vi "Retrieve Airmar Data.vi"(11 "tCRD in":refnum<class "Aircraft OPCCRD.lvclass">) -> (0 "error out":errorcluster, 3 "tCRD out":refnum<class "Aircraft OPCCRD.lvclass">)   [LabVIEW 2015, in "Aircraft OPCCRD.lvclass"]
uses:
  Aircraft OPCCRD.lvclass
  Data/tCRD Data.lvclass
  Reusable/CRDS/Main/CRDS.lvclass
  Reusable/CRDS/Data/Main/CRDS Data.lvclass
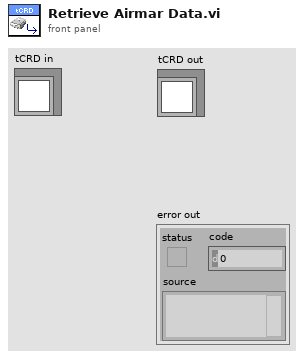
[diagram p1: front panel]
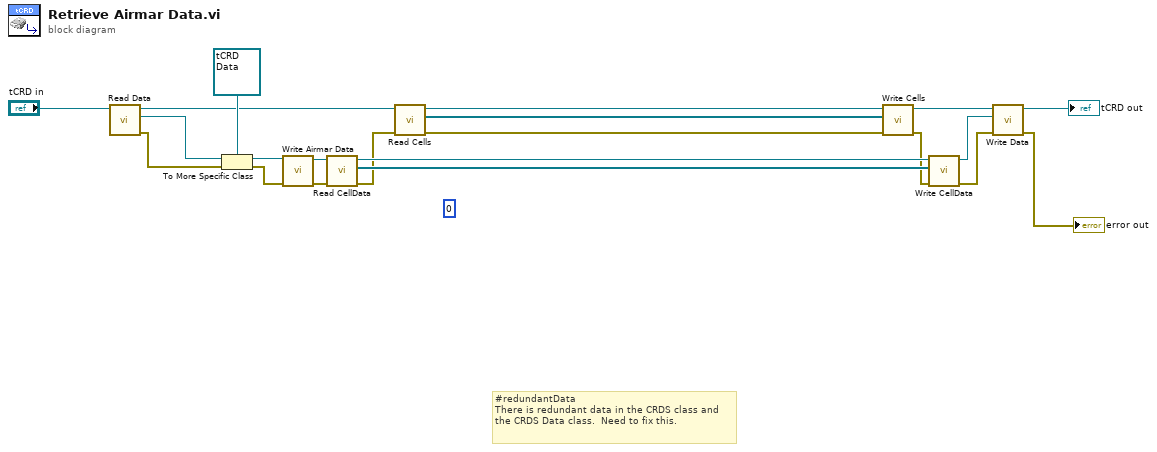
[diagram p0: block diagram]
diagram:
  (unwired) 0
  # "#redundantData\nThere is redundant data in the CRDS class and the CRDS Data class.  Need to fix this."
  n1 = call "Read Data.vi"("CRDS in"="tCRD in") -> ("error out"=w15:errorcluster, "CRDS"=w20:refnum<class "CRDS Data.lvclass">, "CRDS out"=w13:refnum<class "Aircraft OPCCRD.lvclass">, "error in (no error)"=w14:errorcluster)  [unwired: 7 in]
  n2 = To More Specific Class(target class=refnum<class "tCRD Data.lvclass"> refnum ("tCRD Data"), reference=w20, error in=w15) -> (specific class reference=w18:refnum<class "tCRD Data.lvclass">, error out=w17:errorcluster)
  n3 = call "Write Airmar Data.vi"("error in (no error)"=w17, "tCRD Data in"=w18) -> ("error out"=w4:errorcluster, "tCRD Data out"=w8:refnum<class "tCRD Data.lvclass">, "Airmar Data"=w16:refnum<class "Airmar Data.lvclass">)  [unwired: 7 in]
  n4 = call "Read CellData.vi"("error in"=w4, "CRDS Data in"=w8) -> ("error out"=w5:errorcluster, "CellData"=w6:refnum<class "CRDS Cell Data.lvclass">[], "CRDS Data out"=w7:refnum<class "tCRD Data.lvclass">)  [unwired: 7 in]
  n5 = call "Read Cells.vi"("error in (no error)"=w5, "CRDS in"=w13) -> ("error out"=w2:errorcluster, "Cells"=w10:refnum<class "CRDS Cell.lvclass">[], "CRDS out"=w12:refnum<class "Aircraft OPCCRD.lvclass">)  [unwired: 7 in]
  n6 = call "Write Cells.vi"("error in (no error)"=w2, "Cells"=w10, "CRDS in"=w12) -> ("error out"=w1:errorcluster, "CRDS out"=w11:refnum<class "Aircraft OPCCRD.lvclass">)  [unwired: 7 in]
  n7 = call "Write CellData.vi"("error in"=w1, "CellData"=w6, "CRDS Data in"=w7) -> ("error out"=w3:errorcluster, "CRDS Data out"=w9:refnum<class "tCRD Data.lvclass">)  [unwired: 7 in]
  n8 = call "Write Data.vi"("error in (no error)"=w3, "CRDS"=w9, "CRDS in"=w11) -> ("error out"=→"error out":errorcluster, "CRDS out"=→"tCRD out":refnum<class "Aircraft OPCCRD.lvclass">)  [unwired: 7 in]
